vi "SoS_AIR_2025_v1_0_2025.vi"(0 "Temperature":dbl=293.15 format="%.4g", 1 "Frequency":dbl=10.0, 2 "Temperature unit":i32(listbox), 3 "Pressure unit":i32(listbox)=2, 4 "humidity unit":i32(listbox)=3, 5 "frequency unit":i32(listbox)=1, 6 "Humidity":dbl=50.0 format="%.3f", 7 "Type of air":i32(listbox)=4, 8 "Pressure":dbl=1.0 format="%.3f", 9 "CO2 content / ppm":dbl=500.0) -> (11 "Speed of sound rel. st. unc. due to humidity conv. (ppm)":dbl=0.9783901324285029 format="%.1f", 14 "simple speed of sound [m/s]":dbl=344.0424507585898 format="%.4f", 15 "heat capacity corr. speed of sound [m/s]":dbl=343.86139454284574 format="%.4f", 16 "heat capacity & virial corr. speed of sound [m/s]":dbl=343.95466738957066 format="%.4f", 17 "speed of sound humid air  [m/s]":dbl=343.9844045687489 format="%.4f", 18 "Total abs. uncert.":dbl=0.007900284308102695 format="%.4f", 19 "combined rel. st. unc. (ppm)":dbl=22.96698397709987 format="%.1f")   [LabVIEW 2016]
uses:
  SOS_Global_2022.vi
panel:
  out "RH%> 100!":bool
  out "Xw > 1!":bool
  out "heat capacity, virial & relax. corr. speed of sound [m/s]":dbl=343.9844045687489 format="%.4f"
  out "1/2 unc Kr/2 correct 3":dbl=4.518826457384692 format="%.1f"
  out "1/2 relax correction Kr/2 (ppm)":dbl=86.40552705092097 format="%.1f"
  out "1/2 unc Kv/2 correct 2":dbl=22.36531179233521 format="%.1f"
  out "1/2 virial correction Kv/2 (ppm)":dbl=271.28807826462 format="%.1f"
  out "1/2 unc Kc correct":dbl=2.4286089913364837 format="%.1f"
  out "1/2 heat capacity correction Kc/2 (ppm)":dbl=-526.1227906854238 format="%.1f"
  out "Speed of sound rel. st. unc. due to corrections (ppm)":dbl=22.94613487612083 format="%.1f"
  out "relative humidity (%)":dbl=50.0 format="%.3g"
  out "unc Kc correct":dbl=4.857217982672967 format="%.1f"
  out "unc Kv correct":dbl=44.73062358467042
  out "unc Kr correct":dbl=9.037652914769383
  out "enhancement factor":dbl=1.0035661788695114 format="%.6g"
  out "saturation pressure (kPa)":dbl=2.3392491605340155 format="%.3g"
  out "xw Molar fraction H2O":dbl=0.011584462578143766 format="%.6f"
  out "relaxation correction Kr (ppm)":dbl=172.81105410184193 format="%#.0f"
  out "virial correction Kv (ppm)":dbl=542.57615652924
  out "heat capacity correction Kc (ppm)":dbl=-1052.2455813708475
  out "Conversion HR or Tdew --> xw abs. unc.":dbl=6.440526776101253e-06 format="%.6f"
  # "±"
  # "±"
  # "±"
  # "±"
  # "±"
  # "±"
  # "±"
  # "±"
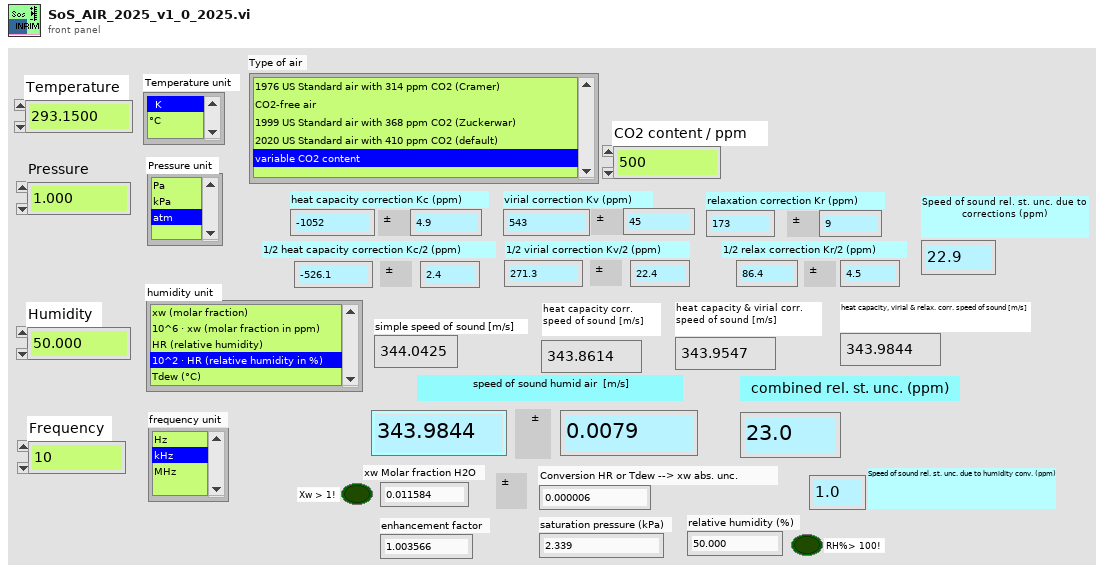
[diagram p1: front panel]
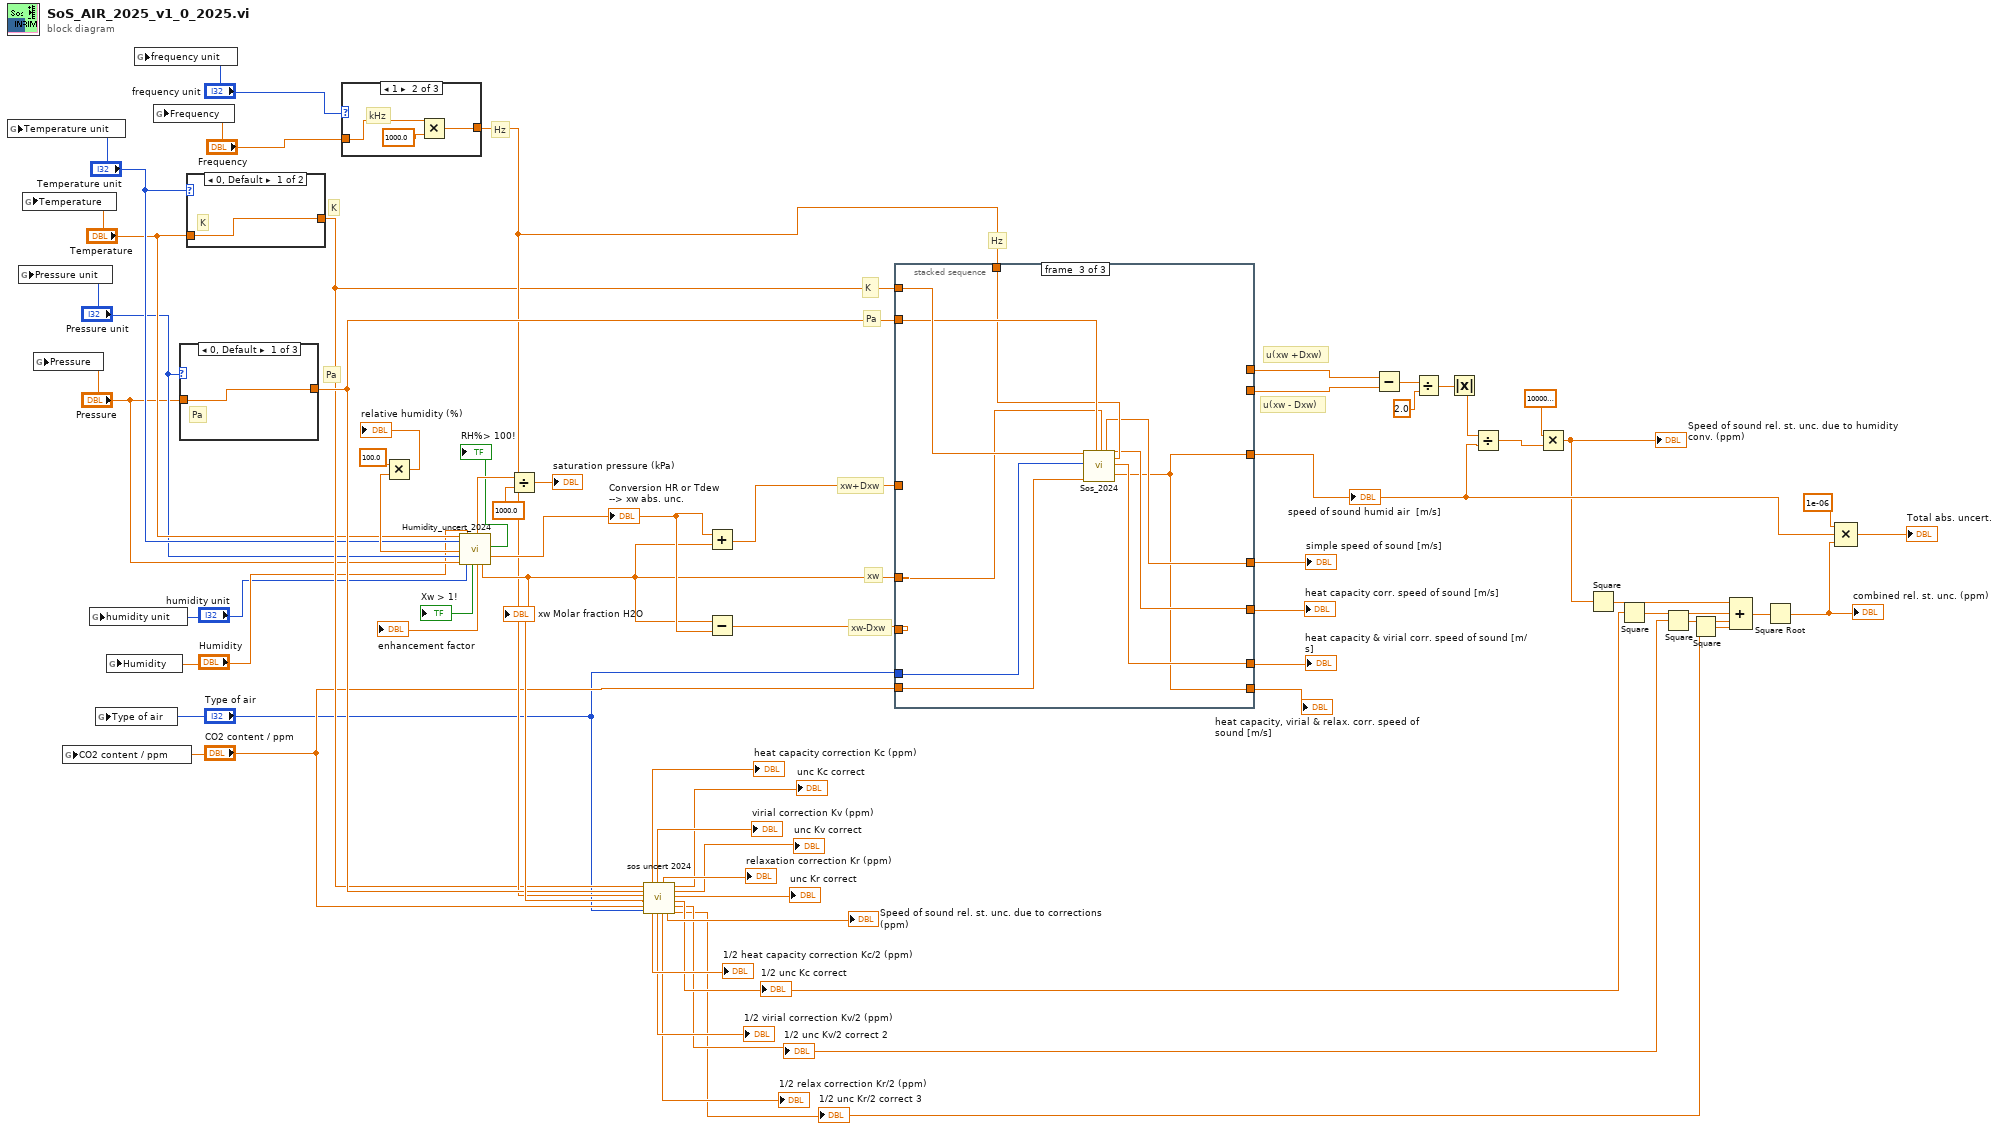
[diagram p0: block diagram]
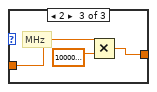
[diagram p3: hidden frame]
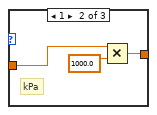
[diagram p4: hidden frame]
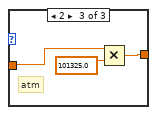
[diagram p5: hidden frame]
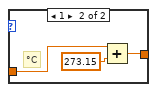
[diagram p6: hidden frame]
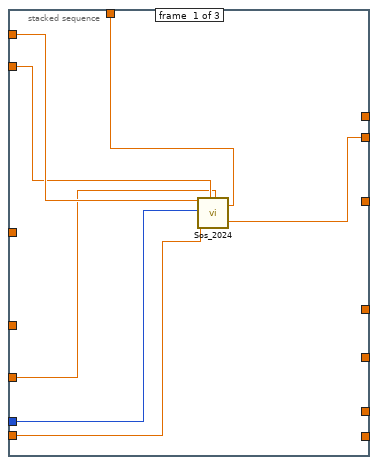
[diagram p7: hidden frame]
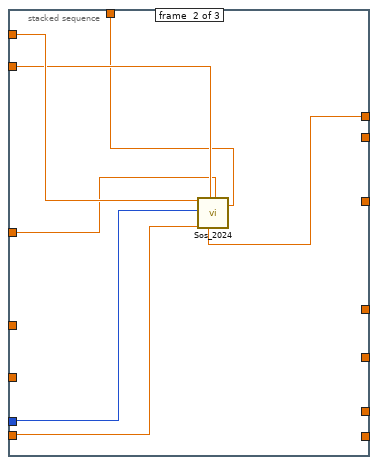
[diagram p8: hidden frame]
diagram:
  # "Hz"
  # "u(xw - Dxw)"
  # "u(xw +Dxw)"
  # "Pa"
  # "K"
  # "xw"
  # "Hz"
  # "xw-Dxw"
  # "Pa"
  # "K"
  # "xw+Dxw"
  n1 = global write "SOS_Global_2022.vi" "Temperature unit"("Temperature unit") -> ()
  n2 = global write "SOS_Global_2022.vi" "Pressure unit"("Pressure unit") -> ()
  n3 = global write "SOS_Global_2022.vi" "Temperature"("Temperature") -> ()
  n4 = global write "SOS_Global_2022.vi" "Pressure"("Pressure") -> ()
  n5 = global write "SOS_Global_2022.vi" "CO2 content / ppm"("CO2 content / ppm") -> ()
  n6 = global write "SOS_Global_2022.vi" "humidity unit"("humidity unit") -> ()
  n7 = global write "SOS_Global_2022.vi" "Type of air"("Type of air") -> ()
  n8 = global write "SOS_Global_2022.vi" "Humidity"("Humidity") -> ()
  n9 = global write "SOS_Global_2022.vi" "frequency unit"("frequency unit") -> ()
  n10 = global write "SOS_Global_2022.vi" "Frequency"("Frequency") -> ()
  n11 = case shown="0, Default" "Pressure unit" {
    tunnel: [w62 w63 w66] -> w29
    tunnel: "Pressure" -> [w62 w64 w67]
    frame 0, Default {
      # "Pa"
    }
    frame 1 {
      # "kPa"
      n12 = Multiply(x=w64, y=1000.0) -> (x*y=w63:dbl)
    }
    frame 2 {
      # "atm"
      n13 = Multiply(x=w67, y=101325.0) -> (x*y=w66:dbl)
    }
  }
  n14 = case shown="0, Default" "Temperature unit" {
    tunnel: [w69 w70] -> w14
    tunnel: "Temperature" -> [w69 w71]
    frame 0, Default {
      # "K"
    }
    frame 1 {
      # "°C"
      n15 = Add(x=w71, y=273.15) -> (x+y=w70:dbl)
    }
  }
  n16 = case shown="1" "frequency unit" {
    tunnel: [w73 w75 w77] -> w28
    tunnel: "Frequency" -> [w73 w76 w78]
    frame 0, Default {
      # "Hz"
    }
    frame 1 {
      # "kHz"
      n17 = Multiply(x=w76, y=1000.0) -> (x*y=w75:dbl)
    }
    frame 2 {
      # "MHz"
      n18 = Multiply(x=w78, y=1000000.0) -> (x*y=w77:dbl)
    }
  }
  n19 = call "Humidity_uncert_2024.vi"("Temperature"="Temperature", "Temperature unit"="Temperature unit", "pressure unit"="Pressure unit", "Pressure"="Pressure", "Humidity"="Humidity", "humidity unit"="humidity unit") -> ("relative humidity"=w45:dbl, "Xw > 1 !"=→"Xw > 1!":bool, "saturation pressure / Pa"=w46:dbl, "enhanc. factor"=→"enhancement factor":dbl, "xw - molar fraction"=w36:dbl, "RH > 1 !"=→"RH%> 100!":bool, "Dxw - molar fraction abs. uncert."=w48:dbl)  [unwired: 1 in, 6 out]
  "Conversion HR or Tdew --> xw abs. unc." <- w48
  "xw Molar fraction H2O" <- w36
  n20 = Multiply(x=100.0, y=w45) -> (x*y=→"relative humidity (%)":dbl)
  n21 = Divide(x=w46, y=1000.0 ("x")) -> (x/y=→"saturation pressure (kPa)":dbl)
  n22 = call "sos uncert 2024.vi"("Temperature / K"=w14, "Pressure / Pa"=w29, "Frequency / Hz"=w28, "xw water molar fraction"=w36, "CO2 content (ppm)"="CO2 content / ppm", "Type of air"="Type of air") -> ("heat capacity correction Kc (ppm)"=→"heat capacity correction Kc (ppm)":dbl, "1/2 heat capacity speed correction Kc/2 (ppm)"=→"1/2 heat capacity correction Kc/2 (ppm)":dbl, "virial correction Kv (ppm)"=→"virial correction Kv (ppm)":dbl, "1/2 virial speed correction Kv/2 (ppm)"=→"1/2 virial correction Kv/2 (ppm)":dbl, "relaxation correction Kr (ppm)"=→"relaxation correction Kr (ppm)":dbl, "1/2 relax speed correction Kr/2 (ppm)"=→"1/2 relax correction Kr/2 (ppm)":dbl, "combined (quadrature sum) relative uncertainty of speed of sound in humid air due to corrections (ppm)"=→"Speed of sound rel. st. unc. due to corrections (ppm)":dbl, "DKc/1+Kc (ppm)"=→"unc Kc correct":dbl, "DKv/1+Kv (ppm)"=→"unc Kv correct":dbl, "DKr/1+Kr (ppm)"=→"unc Kr correct":dbl, "1/2 * DKc/1+Kc - heat capacity rel. uncert. contribution to speed of sound (ppm)"=w17:dbl, "1/2 * DKv/1+Kv - virial rel. uncert. contribution to speed of sound (ppm)"=w16:dbl, "1/2 * DKr/1+Kr - relaxation rel. uncert. contribution to speed of sound (ppm)"=w15:dbl)  [unwired: 1 in]
  "1/2 unc Kc correct" <- w17
  "1/2 unc Kr/2 correct 3" <- w15
  "1/2 unc Kv/2 correct 2" <- w16
  n23 = Add(x=w48, y=w36) -> (x+y=w57:dbl)
  n24 = Subtract(x=w36, y=w48) -> (x-y=w56:dbl)
  n25 = stacked-sequence {
    tunnel: "Type of air" -> [w82 w87 w96]
    tunnel: w14 -> [w86 w93 w103]
    tunnel: w29 -> [w85 w92 w102]
    tunnel: w56 -> [w84 _ _]
    tunnel: w28 -> [w83 w91 w101]
    tunnel: w57 -> [_ w90 _]
    tunnel: [w81 _ _] -> w53
    tunnel: [_ w89 _] -> w49
    tunnel: [_ _ w100] -> w55
    tunnel: [_ _ w99] -> w54
    tunnel: w36 -> [_ _ w98]
    tunnel: [_ _ w94] -> w41
    tunnel: [_ _ w97] -> w52
    tunnel: "CO2 content / ppm" -> [w80 w88 w95]
    tunnel: [_ _ w94] -> w3
    frame #0 {
      n26 = call "Sos_2024.vi"("Temperature (K)"=w86, "Type of air"=w82, "CO2 content (ppm)"=w80, "Pressure (Pa)"=w85, "xw molar fraction water vapor"=w84, "Frequency (Hz)"=w83) -> ("heat & virial & relax corrected speed of sound humid air"=w81:dbl)  [unwired: 7 in, 6 out]
    }
    frame #1 {
      n27 = call "Sos_2024.vi"("Temperature (K)"=w93, "Type of air"=w87, "CO2 content (ppm)"=w88, "Pressure (Pa)"=w92, "xw molar fraction water vapor"=w90, "Frequency (Hz)"=w91) -> ("heat & virial & relax corrected speed of sound humid air"=w89:dbl)  [unwired: 7 in, 6 out]
    }
    frame #2 {
      n28 = call "Sos_2024.vi"("Temperature (K)"=w103, "Type of air"=w96, "CO2 content (ppm)"=w95, "Pressure (Pa)"=w102, "xw molar fraction water vapor"=w98, "Frequency (Hz)"=w101) -> ("simple speed of sound"=w100:dbl, "heat & virial & relax corrected speed of sound humid air"=w94:dbl, "heat capacity corrected speed of sound [m/s]"=w97:dbl, "heat capacity & virial corrected speed of sound"=w99:dbl)  [unwired: 7 in, 3 out]
    }
  }
  "speed of sound humid air  [m/s]" <- w41
  "simple speed of sound [m/s]" <- w55
  "heat capacity corr. speed of sound [m/s]" <- w52
  "heat capacity & virial corr. speed of sound [m/s]" <- w54
  "heat capacity, virial & relax. corr. speed of sound [m/s]" <- w3
  n29 = Subtract(x=w49, y=w53) -> (x-y=w51:dbl)
  n30 = Divide(x=w51, y=2.0) -> (x/y=w44:dbl)
  n31 = Absolute Value(x=w44) -> (abs(x)=w37:dbl)
  n32 = Divide(x=w37, y=w41) -> (x/y=w43:dbl)
  n33 = Multiply(x=1000000.0 ("value"), y=w43) -> (x*y=w26:dbl)
  "Speed of sound rel. st. unc. due to humidity conv. (ppm)" <- w26
  n34 = Square(x=w26) -> (x^2=w25:dbl)
  n35 = Square(x=w17) -> (x^2=w23:dbl)
  n36 = Square(x=w16) -> (x^2=w21:dbl)
  n37 = Square(x=w15) -> (x^2=w19:dbl)
  n38 = Compound Arithmetic op=ADD(w25, w23, w21, w19) -> (w42:dbl)
  n39 = Square Root(x=w42) -> (sqrt(x)=w18:dbl)
  "combined rel. st. unc. (ppm)" <- w18
  n40 = Compound Arithmetic op=MULTIPLY(1e-06 ("value"), w41, w18) -> (→"Total abs. uncert.":dbl)
